vi "MF-101 Industrial Digital Output write DIO.vi"() -> ()   [LabVIEW 8.6]
uses:
  vi.lib/UeiDaq/UeiDaqConfigureTimingForSimpleIO.vi
  <libdir>/resource/objmgr/ueidaq.rc
  vi.lib/UeiDaq/UeiDaqWriteOneDigitalScanUInt16.vi
  vi.lib/UeiDaq/UeiDaqReadOneScaledScan.vi
  vi.lib/UeiDaq/UeiDaqCreateDOIndustrialSession.vi
panel:
  out "raw data decimal":u32[](array[numeric])
  out "Diag Data":dbl[](array[numeric]) format="%#_4g"
  in  "Diagnostic Resource":string
  out "raw data binary":u32[](array[numeric]) format="%b"
  out "Total scans generated":u32
  out "device name":string
  out "DO Resolution (bits)":u32
  in  "Digital Output Resource":string
  in  "DO Port":bool[][](array[boolean])
  out "raw data hex":u32[](array[numeric]) format="%x"
  out "current time":timestamp format="%<%X\n%x>T"
  in  "Refresh rate (ms)":i32
  in  "stop":bool
  # "MF-101 set digital outputs"
  # "1/ Set the resource name -->"
  # "2/ Set the update rate -->"
  # "Diag ch0 = temp_aout0\nDiag ch1 =vsense_p_aout\nDiag ch2 =vsense_n_aout\nDiag ch3 = vdcp_p_aout0\nDiag ch4 =  temp_aout1\nDiag ch5 = vsense_p_aout1\nDiag ch6 = vsense_n_aout1\nDiag ch7 = vdcp_p_aout1\nDiag ch8 = adc_fet0\nDiag ch9 = adc_fet1\nDiag ch10 = adc_fet2\nDiag ch11 = adc_fet3\nDiag ch12 = adc_fet4\nDiag ch13 = adc_fet5\nDiag ch14 = adc_fet6\nDiag ch15 = adc_fet7\nDiag ch16 = adc_fet8\nDiag ch17 = adc_fet9\nDiag ch18 = adc_fet10\nDiag ch19  = adc_fet11\nDiag ch20 = adc_fet12\nDiag ch21 = adc_fet13\nDiag ch22 = adc_fet14\nDiag ch23\t= adc_fet15"
  # "15"
  # "14"
  # "13"
  # "12"
  # "11"
  # "10"
  # "9"
  # "8"
  # "7"
  # "6"
  # "5"
  # "4"
  # "3"
  # "2"
  # "1"
  # "0"
  # "bit 15"
  # "bit 0"
  # "|"
  # "|"
  # "|"
  # "DV 12-15"
  # "DV 8-11"
  # "DV 4-7"
  # "DV 0-3"
  # "voltage applied to DV pins will be switched in/out on selected DO bit"
  # "DO Device info"
  # "-\tDigital FET, specify subsystem 0 in resource string (pdna://192.168.x.x/Devx/DO0/<channels>)   \n   Use DGnd (pins 25, 27, 29, 31) for return"
  # "0"
  # "1"
  # "2"
  # "3"
  # "4"
  # "5"
  # "6"
  # "7"
  # "8"
  # "9"
  # "10"
  # "11"
  # "12"
  # "13"
  # "14"
  # "15"
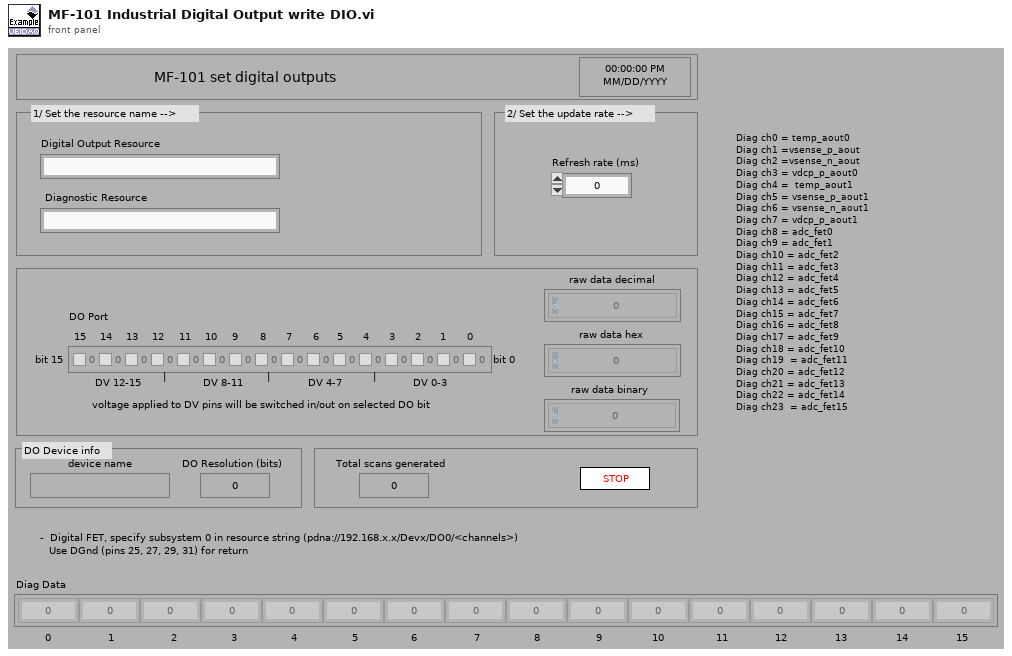
[diagram p1: front panel]
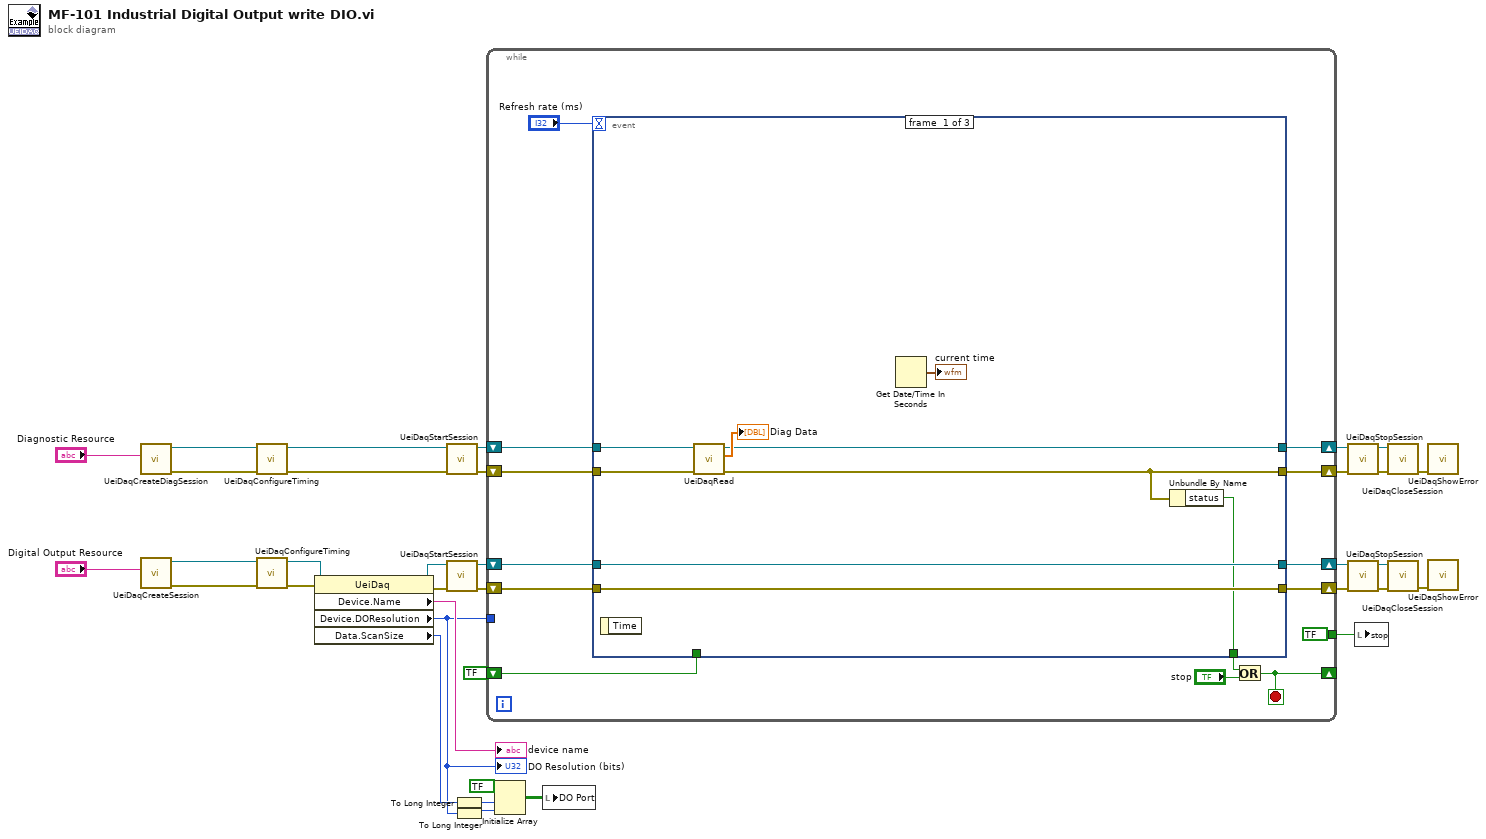
[diagram p0: block diagram]
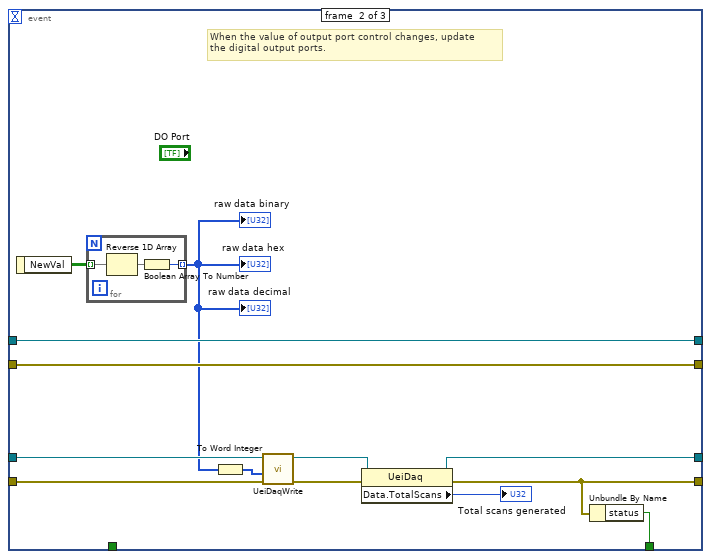
[diagram p2: hidden frame]
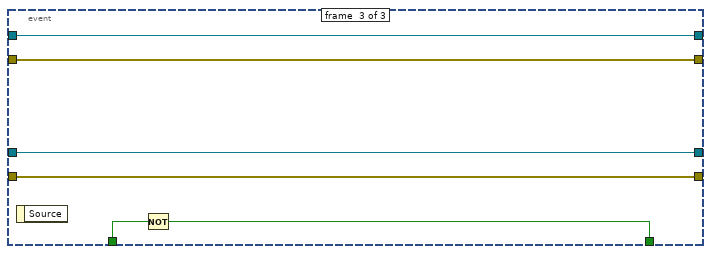
[diagram p3: hidden frame]
diagram:
  n1 = call "UeiDaqCreateDiagSession.vi"("Resource"="Diagnostic Resource") -> ("error out"=w18:errorcluster, "UeiDaq Refnum Out"=w19:refnum<k20>)  [unwired: 9 in]
  n2 = call-poly "UeiDaqCreateSession.vi"("Resource"="Digital Output Resource") -> ("error out"=w33:errorcluster, "UeiDaq Refnum Out"=w34:refnum<k20>)  [unwired: 7 in, 2 out]
  n3 = call-poly "UeiDaqConfigureTiming.vi"("error in (no error)"=w18, "UeiDaq Refnum In"=w19) -> ("error out"=w20:errorcluster, "UeiDaq Refnum Out"=w21:refnum<k20>)  [unwired: 8 out]
  n4 = call-poly "UeiDaqConfigureTiming.vi"("error in (no error)"=w33, "UeiDaq Refnum In"=w34) -> ("error out"=w30:errorcluster, "UeiDaq Refnum Out"=w31:refnum<k20>)  [unwired: 1 in, 7 out]
  n5 = property class="UeiDaq"(reference=w31, error in=w30) -> (reference out=w16:refnum<k20>, error out=w14:errorcluster, "Device.Name"=→"device name":string, "Device.DOResolution"=w23:u32, "Data.ScanSize"=w27:u32)
  "DO Resolution (bits)" <- w23
  n6 = call "UeiDaqStartSession.vi"("error in (no error)"=w20, "UeiDaq Refnum In"=w21) -> ("error out"=w11:errorcluster, "UeiDaq Refnum Out"=w12:refnum<k20>)  [unwired: 8 in]
  n7 = call "UeiDaqStartSession.vi"("error in (no error)"=w14, "UeiDaq Refnum In"=w16) -> ("error out"=w13:errorcluster, "UeiDaq Refnum Out"=w15:refnum<k20>)  [unwired: 8 in]
  n8 = To Long Integer(number=w27) -> (32bit integer=w24:i32)
  n9 = To Long Integer(number=w23) -> (32bit integer=w22:i32)
  n10 = while {
    tunnel: w23 -> [_]
    shift-right: [w41] -> _
    shift-left: bool ? ("x") -> [w44]
    shift-right: [w38] -> w7
    shift-left: w12 -> [w40]
    shift-right: [w37] -> w6
    shift-left: w11 -> [w39]
    shift-right: [w47] -> w5
    shift-left: w15 -> [w49]
    shift-right: [w46] -> w3
    shift-left: w13 -> [w48]
    tunnel: [bool ?] -> w1
    stop <- w41 stop-if-true
    n11 = event shown="[1] \"DO Port\": Value Change" {
      selector: _ -> [_ _ _]
      dyn-events: _ -> [_ _ _]
      timeout: "Refresh rate (ms)" -> [_ _ _]
      tunnel: [w56 w64 w80] -> w46
      tunnel: [w57 w68 w79] -> w47
      tunnel: w49 -> [w57 w70 w79]
      tunnel: w48 -> [w56 w69 w80]
      tunnel: w44 -> [_ _ w78]
      tunnel: [w50 w63 w77] -> w42
      tunnel: w40 -> [w54 w61 w76]
      tunnel: w39 -> [w53 w60 w75]
      tunnel: [w52 w61 w76] -> w38
      tunnel: [w51 w60 w75] -> w37
      event #0 {
        n12 = event-data() -> ()  [unwired: 2 out]
        n13 = call-poly "UeiDaqRead.vi"("error in (no error)"=w53, "UeiDaq Refnum In"=w54) -> ("error out"=w51:errorcluster, "Scaled Data"=→"Diag Data":dbl[], "UeiDaq Refnum Out"=w52:refnum<k20>)  [unwired: 7 in]
        n14 = Get Date/Time In Seconds() -> (seconds since 1Jan1904=→"current time":timestamp)
        n15 = Unbundle By Name(w51) -> ("status"=w50:bool)
      }
      event #1 {
        # "When the value of output port control changes, update\nthe digital output ports."
        n16 = event-data() -> ("NewVal"=w71:bool[][])  [unwired: 1 out]
        n17 = for {
          tunnel: w71 -> [w73] mode=indexing
          tunnel: [w74] -> w59 mode=indexing
          n18 = Reverse 1D Array(array=w73) -> (reversed array=w72:bool[])
          n19 = Boolean Array To Number(Boolean array=w72) -> (number=w74:u32)
        }
        "raw data hex" <- w59
        "raw data binary" <- w59
        "raw data decimal" <- w59
        n20 = To Word Integer(number=w59) -> (16bit integer=w62:i16[])
        n21 = call-poly "UeiDaqWrite.vi"("error in (no error)"=w69, "Digital Data"=w62, "UeiDaq Refnum In"=w70) -> ("error out"=w66:errorcluster, "UeiDaq Refnum Out"=w67:refnum<k20>)  [unwired: 7 out]
        n22 = property class="UeiDaq"(reference=w67, error in=w66) -> (reference out=w68:refnum<k20>, error out=w64:errorcluster, "Data.TotalScans"=→"Total scans generated":u32)
        n23 = Unbundle By Name(w64) -> ("status"=w63:bool)
      }
      event #2 {
        n24 = event-data() -> ()  [unwired: 2 out]
        n25 = Not(x=w78) -> (.not. x?=w77:bool)
      }
    }
    n26 = Or(x=w42, y="stop") -> (x .or. y?=w41:bool)
  }
  n27 = Initialize Array(bool ? ("Boolean"), w24, w22) -> (w28:bool[][])
  n28 = local write "DO Port"(w28) -> ()
  n29 = call "UeiDaqStopSession.vi"("error in (no error)"=w6, "UeiDaq Refnum In"=w7) -> ("error out"=w8:errorcluster, "UeiDaq Refnum Out"=w9:refnum<k20>)  [unwired: 8 in]
  n30 = call "UeiDaqStopSession.vi"("error in (no error)"=w3, "UeiDaq Refnum In"=w5) -> ("error out"=w2:errorcluster, "UeiDaq Refnum Out"=w4:refnum<k20>)  [unwired: 8 in]
  n31 = local write "stop"(w1) -> ()
  n32 = call "UeiDaqCloseSession.vi"("error in (no error)"=w8, "UeiDaq Refnum In"=w9) -> ("error out"=w10:errorcluster)  [unwired: 1 in, 8 out]
  n33 = call "UeiDaqCloseSession.vi"("error in (no error)"=w2, "UeiDaq Refnum In"=w4) -> ("error out"=w35:errorcluster)  [unwired: 1 in, 8 out]
  n34 = call "UeiDaqShowError.vi"("error in (no error)"=w10) -> ()  [unwired: 2 in, 9 out]
  n35 = call "UeiDaqShowError.vi"("error in (no error)"=w35) -> ()  [unwired: 2 in, 9 out]
